vi "ConfigAI_RC.vi"(3 "Task out":tag, 8 "error in":errorcluster, 9 "DAQmx Channel Specs":T2(array[cluster]) {"Max value" min=0.0 max=10.0 step=1.0; "Min value" min=-10.0 max=10.0 step=1.0}, 11 "DAQ params":T1 {"Trigger slope" items=["Rising", "Falling"]; "Trigger level" min=-10.0 max=10.0 step=1.0 scale=-10.0..10.0}) -> (0 "error out":errorcluster)   [LabVIEW 2023]
uses:
  DAQmxParams.ctl
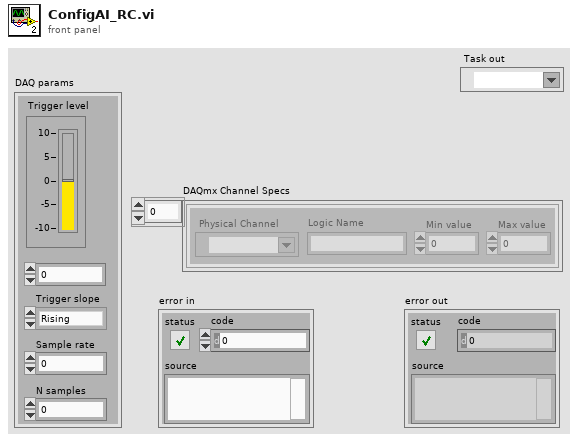
[diagram p1: front panel]
types:
  T1 = typedef "DAQmxParams.ctl" = cluster{"Trigger level":dbl, "Trigger slope":u16, "Sample rate":dbl, "N samples":i32}
  T2 = cluster{" Physical Channel":tag, "Logic Name":string, "Min value":dbl, "Max value":dbl}[]
  T3 = cluster{" Physical Channel":tag, "Logic Name":string, "Min value":dbl, "Max value":dbl}
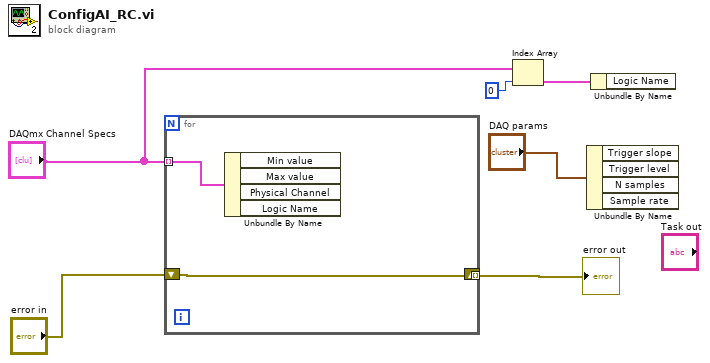
[diagram p0: block diagram]
diagram:
  n1 = for {
    tunnel: "DAQmx Channel Specs" -> [w8] mode=indexing
    tunnel: [w7] -> w2 mode=indexing
    shift-right: _ -> [_]
    shift-left: "error in" -> [w7]
    n2 = Unbundle By Name(w8) -> ()  [unwired: 4 out]
  }
  "error out" <- w2
  n3 = Index Array(array="DAQmx Channel Specs", index=0) -> (element=w5:T3)
  n4 = Unbundle By Name("DAQ params") -> ()  [unwired: 4 out]
  n5 = Unbundle By Name(w5) -> ()  [unwired: 1 out]
